vi "ApplySpectrometerSettings.vi"(8 "error in (no error)":errorcluster, 11 "StellarNetSpecAcquisition in":refnum<class "StellarNetSpecAcquisition.lvclass">) -> (0 "error out":errorcluster, 3 "StellarNetSpecAcquisition out":refnum<class "StellarNetSpecAcquisition.lvclass">)   [LabVIEW 2013, in "StellarNetSpecAcquisition.lvclass"]
uses:
  StellarNetSpecAcquisition.lvclass
  StellarNetSpecAcquisition.lvclass/StellarNetSpecAcquisition.ctl
  StellarNetSpectrometerClass/StellarNetSpectrometer.lvclass
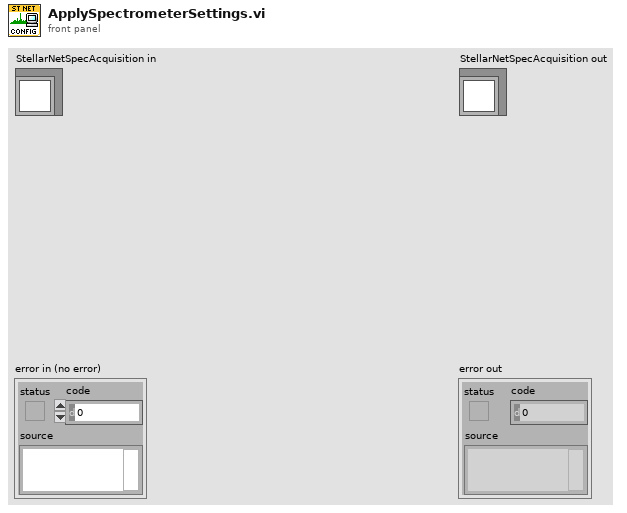
[diagram p1: front panel]
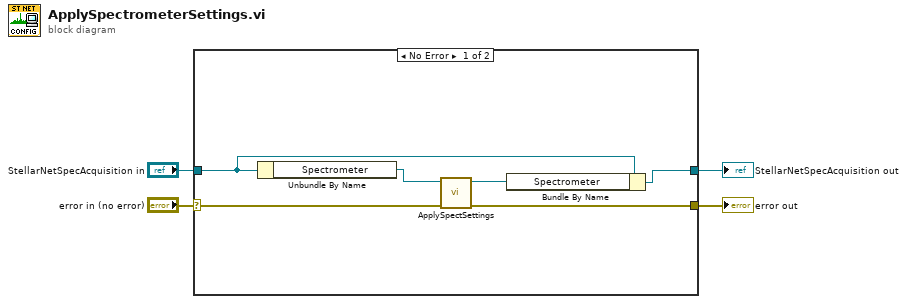
[diagram p0: block diagram]
diagram:
  n1 = case shown="No Error" "error in (no error)" {
    selector: "error in (no error)" -> [w9 w12]
    tunnel: [w8 w12] -> w3
    tunnel: [w6 w11] -> w1
    tunnel: "StellarNetSpecAcquisition in" -> [w7 w11]
    frame No Error {
      n2 = Unbundle By Name(w7) -> ("Spectrometer"=w10:refnum<class "StellarNetSpectrometer.lvclass">)
      n3 = call-dynamic "ApplySpectSettings.vi"("error in"=w9, "StellarNetSpectrometer in"=w10) -> ("error out"=w8:errorcluster, "StellarNetSpectrometer out"=w5:refnum<class "StellarNetSpectrometer.lvclass">)  [unwired: 8 in]
      n4 = Bundle By Name(cluster=w7, "Spectrometer"=w5) -> (w6:refnum<class "StellarNetSpecAcquisition.lvclass">)
    }
    frame Error {
    }
  }
  "error out" <- w3
  "StellarNetSpecAcquisition out" <- w1
